vi "Get Lifecycle State.vi"(8 "error in (no error)":errorcluster, 11 "Process In":refnum<class "Process.lvclass">) -> (0 "error out":errorcluster, 1 "API Mode":T1, 2 "Lifecycle State":T2, 3 "Process Out":refnum<class "Process.lvclass">)   [LabVIEW 2020, in "Process.lvclass"]
doc: "Returns the current life cycle state of the process. \n\nThe API Mode is used to determine if this VI is called from within the process loop or from outside. If called from outside, a message should be sent to the process loop where it may be handled. If called from inside the process loop, the message should be handled and message passing should be avoided.\n\nThe enum replaced earlier implementations, using a boolean flag, to make code more self documenting. The logic remains unchanged and the change is unbroken."
uses:
  Process.lvclass
  Lifecycle State.ctl
  Process.lvclass/Process.ctl
  API Mode.ctl
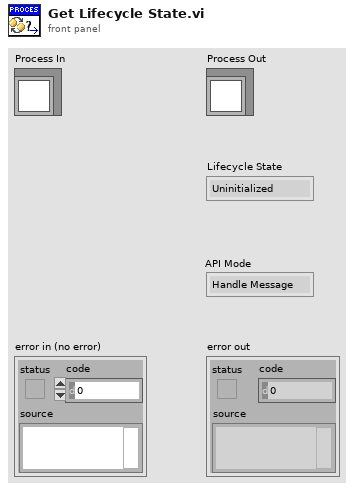
[diagram p1: front panel]
types:
  T1 = typedef "Process.lvclass/API Mode.ctl" = enum16{"Handle Message", "Send Message"}
  T2 = typedef "Process.lvclass/Lifecycle State.ctl" = enum16{"Uninitialized", "Initialized", "Started", "Running", "Stopped", "Finished"}
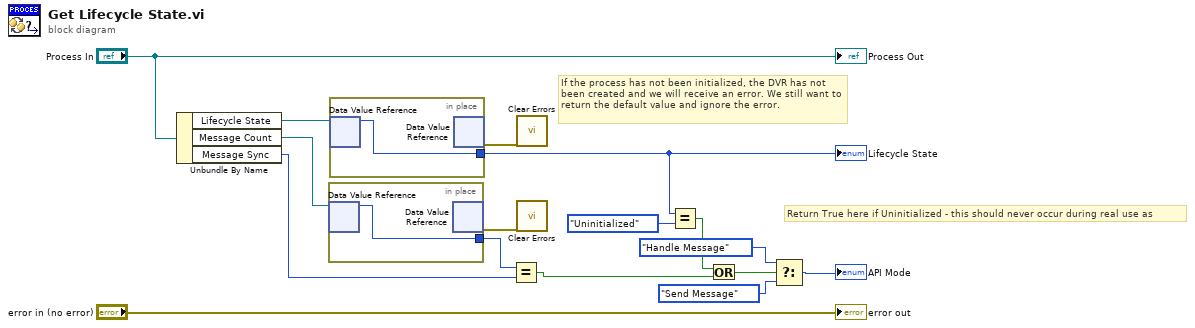
[diagram p0: block diagram]
diagram:
  # "Return True here if Uninitialized - this should never occur during real use as"
  # "If the process has not been initialized, the DVR has not been created and we will receive an error. We still want to return the default value and ignore the error."
  n1 = Unbundle By Name("Process In") -> ("Lifecycle State"=w15:refnum<data-value>, "Message Count"=w12:refnum<data-value>, "Message Sync"=w10:i32)
  n2 = in-place {
    in-place-border: [w17] -> w11
    n3 = in-place-dvr #1(w12) -> (w17:i32)  [unwired: 1 out]
    n4 = in-place-dvr #1() -> (w8:errorcluster)  [unwired: 1 in, 1 out]
  }
  n5 = in-place {
    in-place-border: [w18] -> w7
    n6 = in-place-dvr #2(w15) -> (w18:T2)  [unwired: 1 out]
    n7 = in-place-dvr #2() -> (w13:errorcluster)  [unwired: 1 in, 1 out]
  }
  "Lifecycle State" <- w7
  n8 = Equal?(x=w11, y=w10) -> (x = y?=w9:bool)
  n9 = call <vilib>:"Clear Errors.vi"("error in (no error)"=w13) -> ()  [unwired: 5 in, 2 out]
  n10 = call <vilib>:"Clear Errors.vi"("error in (no error)"=w8) -> ()  [unwired: 5 in, 2 out]
  n11 = Equal?(x=w7, y=Lifecycle_State."Uninitialized") -> (x = y?=w5:bool)
  n12 = Or(x=w5, y=w9) -> (x .or. y?=w4:bool)
  n13 = Select(t=API_Mode."Handle Message" ("API Mode"), s=w4, f=API_Mode."Send Message" ("API Mode")) -> (s? t:f=→"API Mode":T1)
  "error out" <- "error in (no error)"
  "Process Out" <- "Process In"
